vi "HysteresisCompensationWithOptimization.vi"() -> ()   [LabVIEW 2016]
uses:
  controls/Enum.ctl
  <vilib>/gmath/NumericalOptimization/stopping criteria.ctl
  <vilib>/gmath/NumericalOptimization/conjugate gradient settings.ctl
  <vilib>/gmath/NumericalOptimization/ucno_user objective function ref.ctl
  <vilib>/Utility/file.llb/Write Delimited Spreadsheet (DBL).vi
  <vilib>/gmath/NumericalOptimization/Conjugate Gradient.vi
  <vilib>/gmath/NI_Gmath.lvlib
panel:
  in  "Save":bool
  in  "Calculate":bool
  in  "Direction":enum16{"Fast", "Slow"}(ring)
  in  "Polynom order":i32=4
  out "corrected":dbl[][](graph)
  out "uncorrected":sgl[][](graph)
  out "error out":errorcluster
  out "number of function evaluations":i32
  out "f(minimum)":dbl
  out "minimum":dbl[](array[numeric])
  # "Run this VI after having scanned several lines and the scan is stopped or paused. The Scan Waveform should not be Hysteresis Compensated.\nIt will calculate the polynomial coefficients correcting the hysteresis and send it to the FGV read in ScanWaveforms.vi.\nIn ScanWaveform, update the hysteresis and update the FPGA."
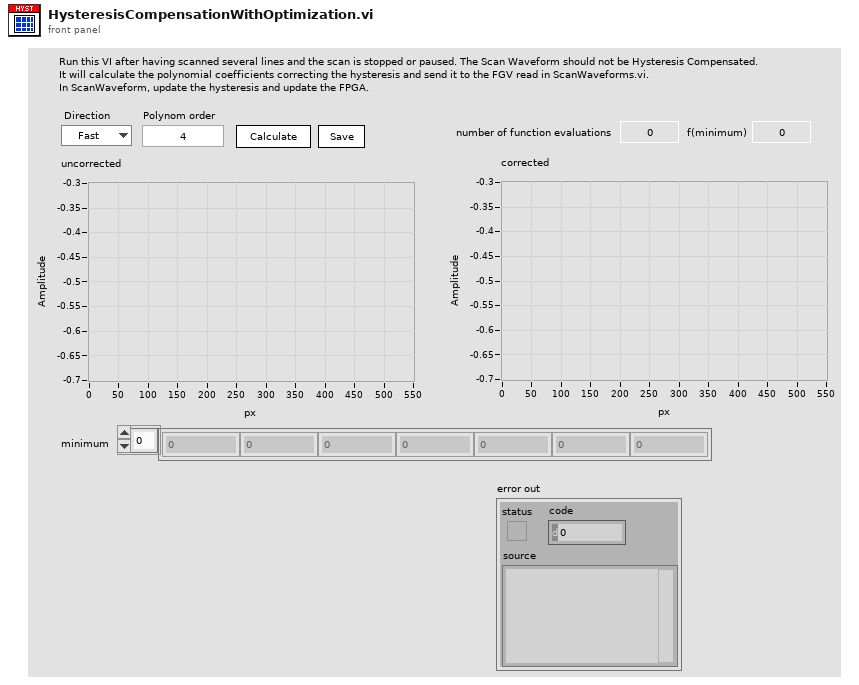
[diagram p1: front panel]
types:
  T1 = typedef "NI_Gmath.lvlib/stopping criteria.ctl" = cluster{"function tolerance":dbl, "parameter tolerance":dbl, "max iterations":i32, "max function calls":i32, "gradient tolerance":dbl, "max time (sec)":dbl}
  T2 = typedef "NI_Gmath.lvlib/conjugate gradient settings.ctl" = cluster{"gradient method":enum16{"Fletcher-Reeves", "Polak-Ribiere"}, "line minimization":enum16{"without derivatives", "with derivatives"}}
  T3 = typedef "Enum.ctl" = enum16{"Init", "Read", "Write"}
  T4 = typedef "NI_Gmath.lvlib/ucno_user objective function ref.ctl" = refnum<vi>
  T5 = cluster{"CorrectionToFGV":bool, "PolynomCoeff":dbl[], "CorrectionToFPGA":bool}
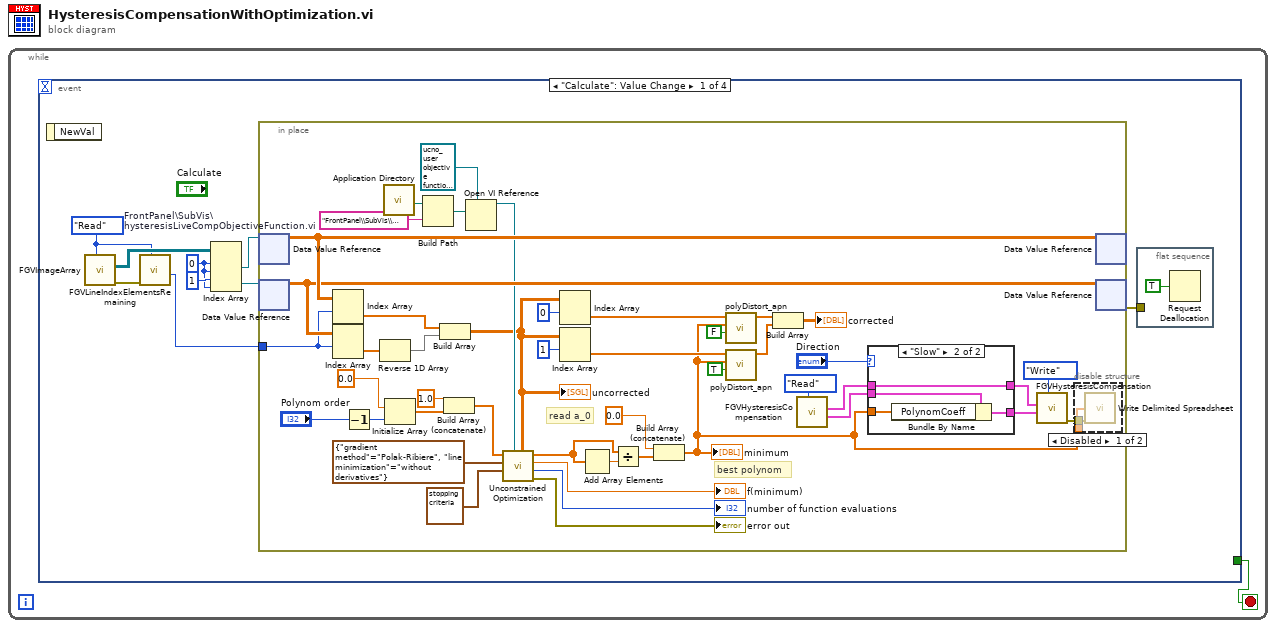
[diagram p0: block diagram]
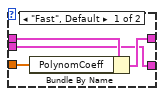
[diagram p3: hidden frame]
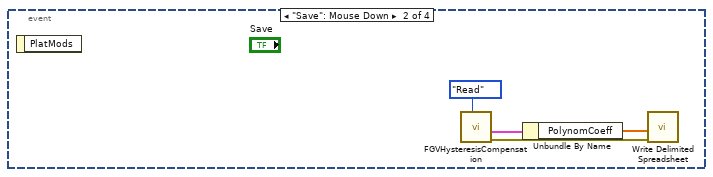
[diagram p4: hidden frame]
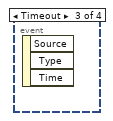
[diagram p5: hidden frame]
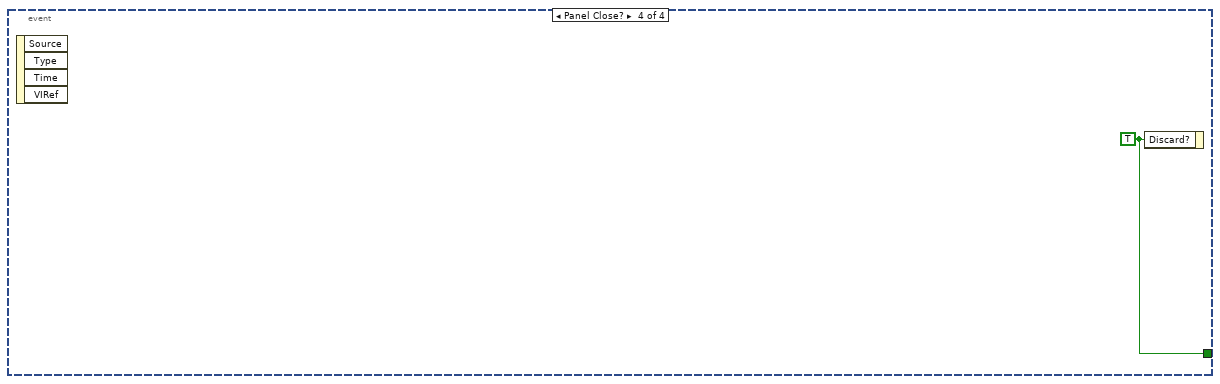
[diagram p6: hidden frame]
diagram:
  n1 = while {
    stop <- w1 stop-if-true
    n2 = event shown="[0] \"Calculate\": Value Change" {
      selector: _ -> [_ _ _ _]
      dyn-events: _ -> [_ _ _ _]
      timeout: _ -> [_ _ _ _]
      tunnel: [_ _ _ w71] -> w1
      event "Calculate": Value Change {
        w7 = 0 ("disabled index (page)")
        w2 = Enum."Read" ("Enum")
        n3 = event-data() -> ()  [unwired: 1 in, 1 out]
        n4 = call "FGVImageArray.vi"("Enum"=w2) -> ("error out"=w9:errorcluster, "ImageRefOut"=w6:refnum<data-value>[][])  [unwired: 9 in]
        n5 = call "FGVLineIndexElementsRemaining.vi"("Enum"=w2, "error in"=w9) -> ("lineIndexOut"=w3:u32)  [unwired: 8 in, 1 out]
        n6 = Index Array(array=w6, index (row) #1=w7, index (col) #1=w7, index (row) #2=1 ("disabled index (vol)"), index (col) #2=w7) -> (element #1=w5:refnum<data-value>, element #2=w4:refnum<data-value>)
        n7 = in-place {
          in-place-border: w3 -> [w14]
          w36 = "FrontPanel\\SubVis\\hysteresisLiveCompObjectiveFunction.vi"  # FrontPanel\SubVis\hysteresisLiveCompObjectiveFunction.vi
          # "best polynom"
          # "read a_0"
          n8 = in-place-dvr #1(w5) -> (w55:sgl[][])  [unwired: 1 out]
          n9 = in-place-dvr #2(w4) -> (w54:sgl[][])  [unwired: 1 out]
          n10 = Index Array(array=w55, index (row)=w14) -> (element=w51:sgl[])  [unwired: 1 in]
          n11 = Index Array(array=w54, index (row)=w14) -> (element=w53:sgl[])  [unwired: 1 in]
          n12 = Decrement(x="Polynom order") -> (x-1=w44:i32)
          n13 = Reverse 1D Array(array=w53) -> (reversed array=w52:sgl[])
          n14 = call <vilib>:"Application Directory.vi"() -> ("Application Directory"=w35:path)
          n15 = Initialize Array(0.0 ("element"), w44) -> (w43:dbl[])
          n16 = Build Path(base path=w35, name or relative path=w36) -> (appended path=w37:path)
          n17 = Build Array(w51, w52) -> (w13:sgl[][])
          "uncorrected" <- w13
          n18 = Build Array (concatenate)(1.0 ("element"), w43) -> (w40:dbl[])
          n19 = Open VI Reference(type specifier VI Refnum (for type only)=T4 refnum ("objective function"), vi path=w37) -> (vi reference=w21:T4)  [unwired: 4 in, 1 out]
          n20 = call-poly <vilib>:"Unconstrained Optimization.vi"("function data"=w13, "objective function"=w21, "stopping criteria"=T1 {"function tolerance"=0.1, "parameter tolerance"=1e-05, "max iterations"=1000, "max function calls"=10000, "gradient tolerance"=1e-07, "max time (sec)"=10.0}, "conjugate gradient settings"=T2 {"gradient method"=enum."Polak-Ribiere", "line minimization"=enum."without derivatives"}, "start"=w40) -> ("error out"=→"error out":errorcluster, "number of function evaluations"=→"number of function evaluations":i32, "f(minimum)"=→"f(minimum)":dbl, "minimum"=w32:dbl[])  [unwired: 3 in]
          n21 = Index Array(array=w13, index (row)=0) -> (element=w24:sgl[])  [unwired: 1 in]
          n22 = Index Array(array=w13, index (row)=1) -> (element=w25:sgl[])  [unwired: 1 in]
          n23 = Add Array Elements(numeric array=w32) -> (sum=w31:dbl)
          n24 = Divide(x=w32, y=w31) -> (x/y=w33:dbl[])
          n25 = Build Array (concatenate)(0.0, w33) -> (w11:dbl[])
          "minimum" <- w11
          n26 = call "polyDistort_apn.vi"("Backward?"=FALSE, "polyIn"=w11, "lineDataIn"=w24) -> ("distoredDataOut"=w28:dbl[])  [unwired: 7 in, 1 out]
          n27 = call "polyDistort_apn.vi"("Backward?"=TRUE, "polyIn"=w11, "lineDataIn"=w25) -> ("distoredDataOut"=w29:dbl[])  [unwired: 7 in, 1 out]
          n28 = Build Array(w28, w29) -> (→"corrected":dbl[][])
          n29 = call "FGVHysteresisCompensation.vi"("Enum"=Enum."Read") -> ("HysteresisSlowOut"=w46:T5, "HysteresisFastOut"=w45:T5)  [unwired: 8 in, 1 out]
          n30 = case shown="\"Slow\"" "Direction" {
            tunnel: w45 -> [w60 w62]
            tunnel: w46 -> [w58 w64]
            tunnel: w11 -> [w61 w65]
            tunnel: [w58 w63] -> w49
            tunnel: [w59 w62] -> w50
            frame "Fast", Default {
              n31 = Bundle By Name(cluster=w60, "PolynomCoeff"=w61) -> (w59:T5)
            }
            frame "Slow" {
              n32 = Bundle By Name(cluster=w64, "PolynomCoeff"=w65) -> (w63:T5)
            }
          }
          n33 = call "FGVHysteresisCompensation.vi"("Enum"=Enum."Write", "HysteresisSlowIn"=w49, "HysteresisFastIn"=w50) -> ("error out"=w12:errorcluster)  [unwired: 6 in, 2 out]
          n34 = disable-structure shown="Disabled" {
            disable-tunnel: w12 -> [w57 _]
            disable-tunnel: w11 -> [w56 _]
            frame Disabled {
              n35 = call-poly <vilib>:"Write Delimited Spreadsheet.vi"("1D data"=w56, "error in (no error)"=w57) -> ()  [unwired: 12 in, 2 out]
            }
            frame Enabled {
            }
          }
          n36 = in-place-dvr #1(w55) -> ()  [unwired: 2 out]
          n37 = in-place-dvr #2(w54) -> (w10:errorcluster)  [unwired: 1 out]
        }
        n38 = flat-sequence {
          tunnel: w10 -> [_]
          frame #0 {
            n39 = Request Deallocation(TRUE ("flag")) -> ()
          }
        }
      }
      event "Save": Mouse Down {
        n40 = event-data() -> ()  [unwired: 1 in, 1 out]
        n41 = call "FGVHysteresisCompensation.vi"("Enum"=Enum."Read") -> ("error out"=w69:errorcluster, "HysteresisSlowOut"=w68:T5)  [unwired: 8 in, 1 out]
        n42 = Unbundle By Name(w68) -> ("PolynomCoeff"=w67:dbl[])
        n43 = call-poly <vilib>:"Write Delimited Spreadsheet.vi"("1D data"=w67, "error in (no error)"=w69) -> ()  [unwired: 12 in, 2 out]
      }
      event Timeout {
        n44 = event-data() -> ()  [unwired: 1 in, 3 out]
      }
      event Panel Close? {
        w71 = TRUE ("Discard?")
        n45 = event-data() -> ()  [unwired: 1 in, 4 out]
        n46 = event-data("Discard?"=w71) -> ()  [unwired: 1 in, 1 out]
      }
    }
  }
